vi "TEMP.vi"(8 "error in (no error)":errorcluster caption="error in", 10 "Temperature":dbl format="%.2f", 11 "Camera Handle":u32) -> (0 "error out":errorcluster, 1 "String":string, 2 "INI Flag":bool, 3 "Camera Handle":u32)   [LabVIEW 2015]
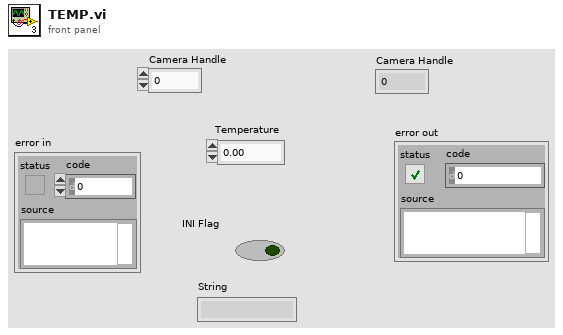
[diagram p1: front panel]
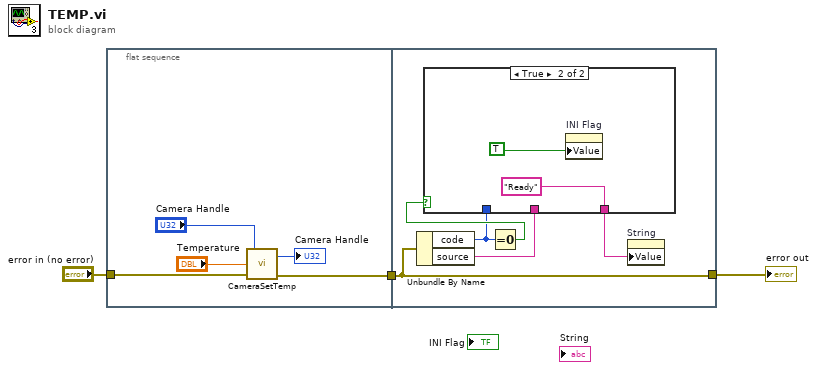
[diagram p0: block diagram]
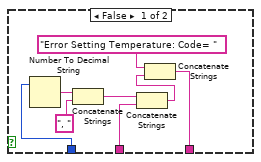
[diagram p2: hidden frame]
diagram:
  n1 = flat-sequence {
    tunnel: [w8] -> w3
    tunnel: "error in (no error)" -> [w7]
    tunnel: w3 -> [w13]
    tunnel: [w13] -> w1
    frame #0 {
      n2 = call <userlib>:"CameraSetTemp.vi"("error in (no error)"=w7, "Temperature"="Temperature", "Camera Handle"="Camera Handle") -> ("error out"=w8:errorcluster, "Camera Handle"=→"Camera Handle":u32)
    }
    frame #1 {
      n3 = Unbundle By Name(w13) -> ("code"=w10:i32, "source"=w11:string)
      n4 = Equal To 0?(x=w10) -> (x = 0?=w12:bool)
      n5 = case shown="True" w12 {
        tunnel: [w14 "Ready"] -> w9
        tunnel: w11 -> [w15 _]
        tunnel: w10 -> [w20 _]
        frame False {
          n6 = Number To Decimal String(number=w20) -> (decimal integer string=w19:string)  [unwired: 1 in]
          n7 = Concatenate Strings(w19, ", ") -> (w16:string)
          n8 = Concatenate Strings(w16, w15) -> (w17:string)
          n9 = Concatenate Strings("Error Setting Temperature: Code= ", w17) -> (w14:string)
        }
        frame True {
          n10 = property on="INI Flag" class="Bool (strict)"("Value"=TRUE) -> ()  [unwired: 2 in, 2 out]
        }
      }
      n11 = property on="String" class="Str"("Value"=w9) -> ()  [unwired: 2 in, 2 out]
    }
  }
  "error out" <- w1
